vi "Strip Path Extension__ogtk.vi"   [LabVIEW 2020]
doc: "Splits a relative or absolute path into its root and extension. Path can be a string, path, or array of strings or paths.\nFor example:\n\npath => c:\\temp\\lock.txt\nroot => \"c:\\temp\\lock\"\nextension => \"txt\"\n\npath => temp\\lock.txt\nroot => \"temp\\lock\"\nextension => \"txt\"\n\npath => c:\\temp.folder\\lock\nroot => \"c:\\temp.folder\\lock\"\nextension => \"\"\n\npath => lock.txt\nroot => \"lock\"\nextension => \"txt\""
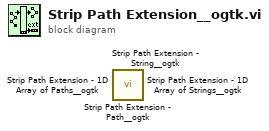
[diagram p0: block diagram]
diagram:
  n1 = call <userlib>:"Strip Path Extension - Path__ogtk.vi"() -> ()  [unwired: 1 in, 2 out]
  n2 = call <userlib>:"Strip Path Extension - String__ogtk.vi"() -> ()  [unwired: 1 in, 2 out]
  n3 = call <userlib>:"Strip Path Extension - 1D Array of Paths__ogtk.vi"() -> ()  [unwired: 1 in, 2 out]
  n4 = call <userlib>:"Strip Path Extension - 1D Array of Strings__ogtk.vi"() -> ()  [unwired: 1 in, 2 out]
